vi "run_control.vi"() -> ()   [LabVIEW 2011]
panel:
  out "error out":errorcluster
  out "Last Remote Port":i64
  out "Last Remote Address":string
  out "Connection Msg":errorcluster
  out "Real-time Data from PLCs (Actuation)":string[][](array[string])
  out "# of data":i32
  out "# of data":i32
  out "# of data":i32
  out "# of data":i32
  out "# of received data":u64
  out "Real-time Data from People Counter":string[][](array[string])
  out "Real-time Data from PLCs (Sensing)":string[][](array[string])
  out "Real-time Data from Motes":string[][](array[string])
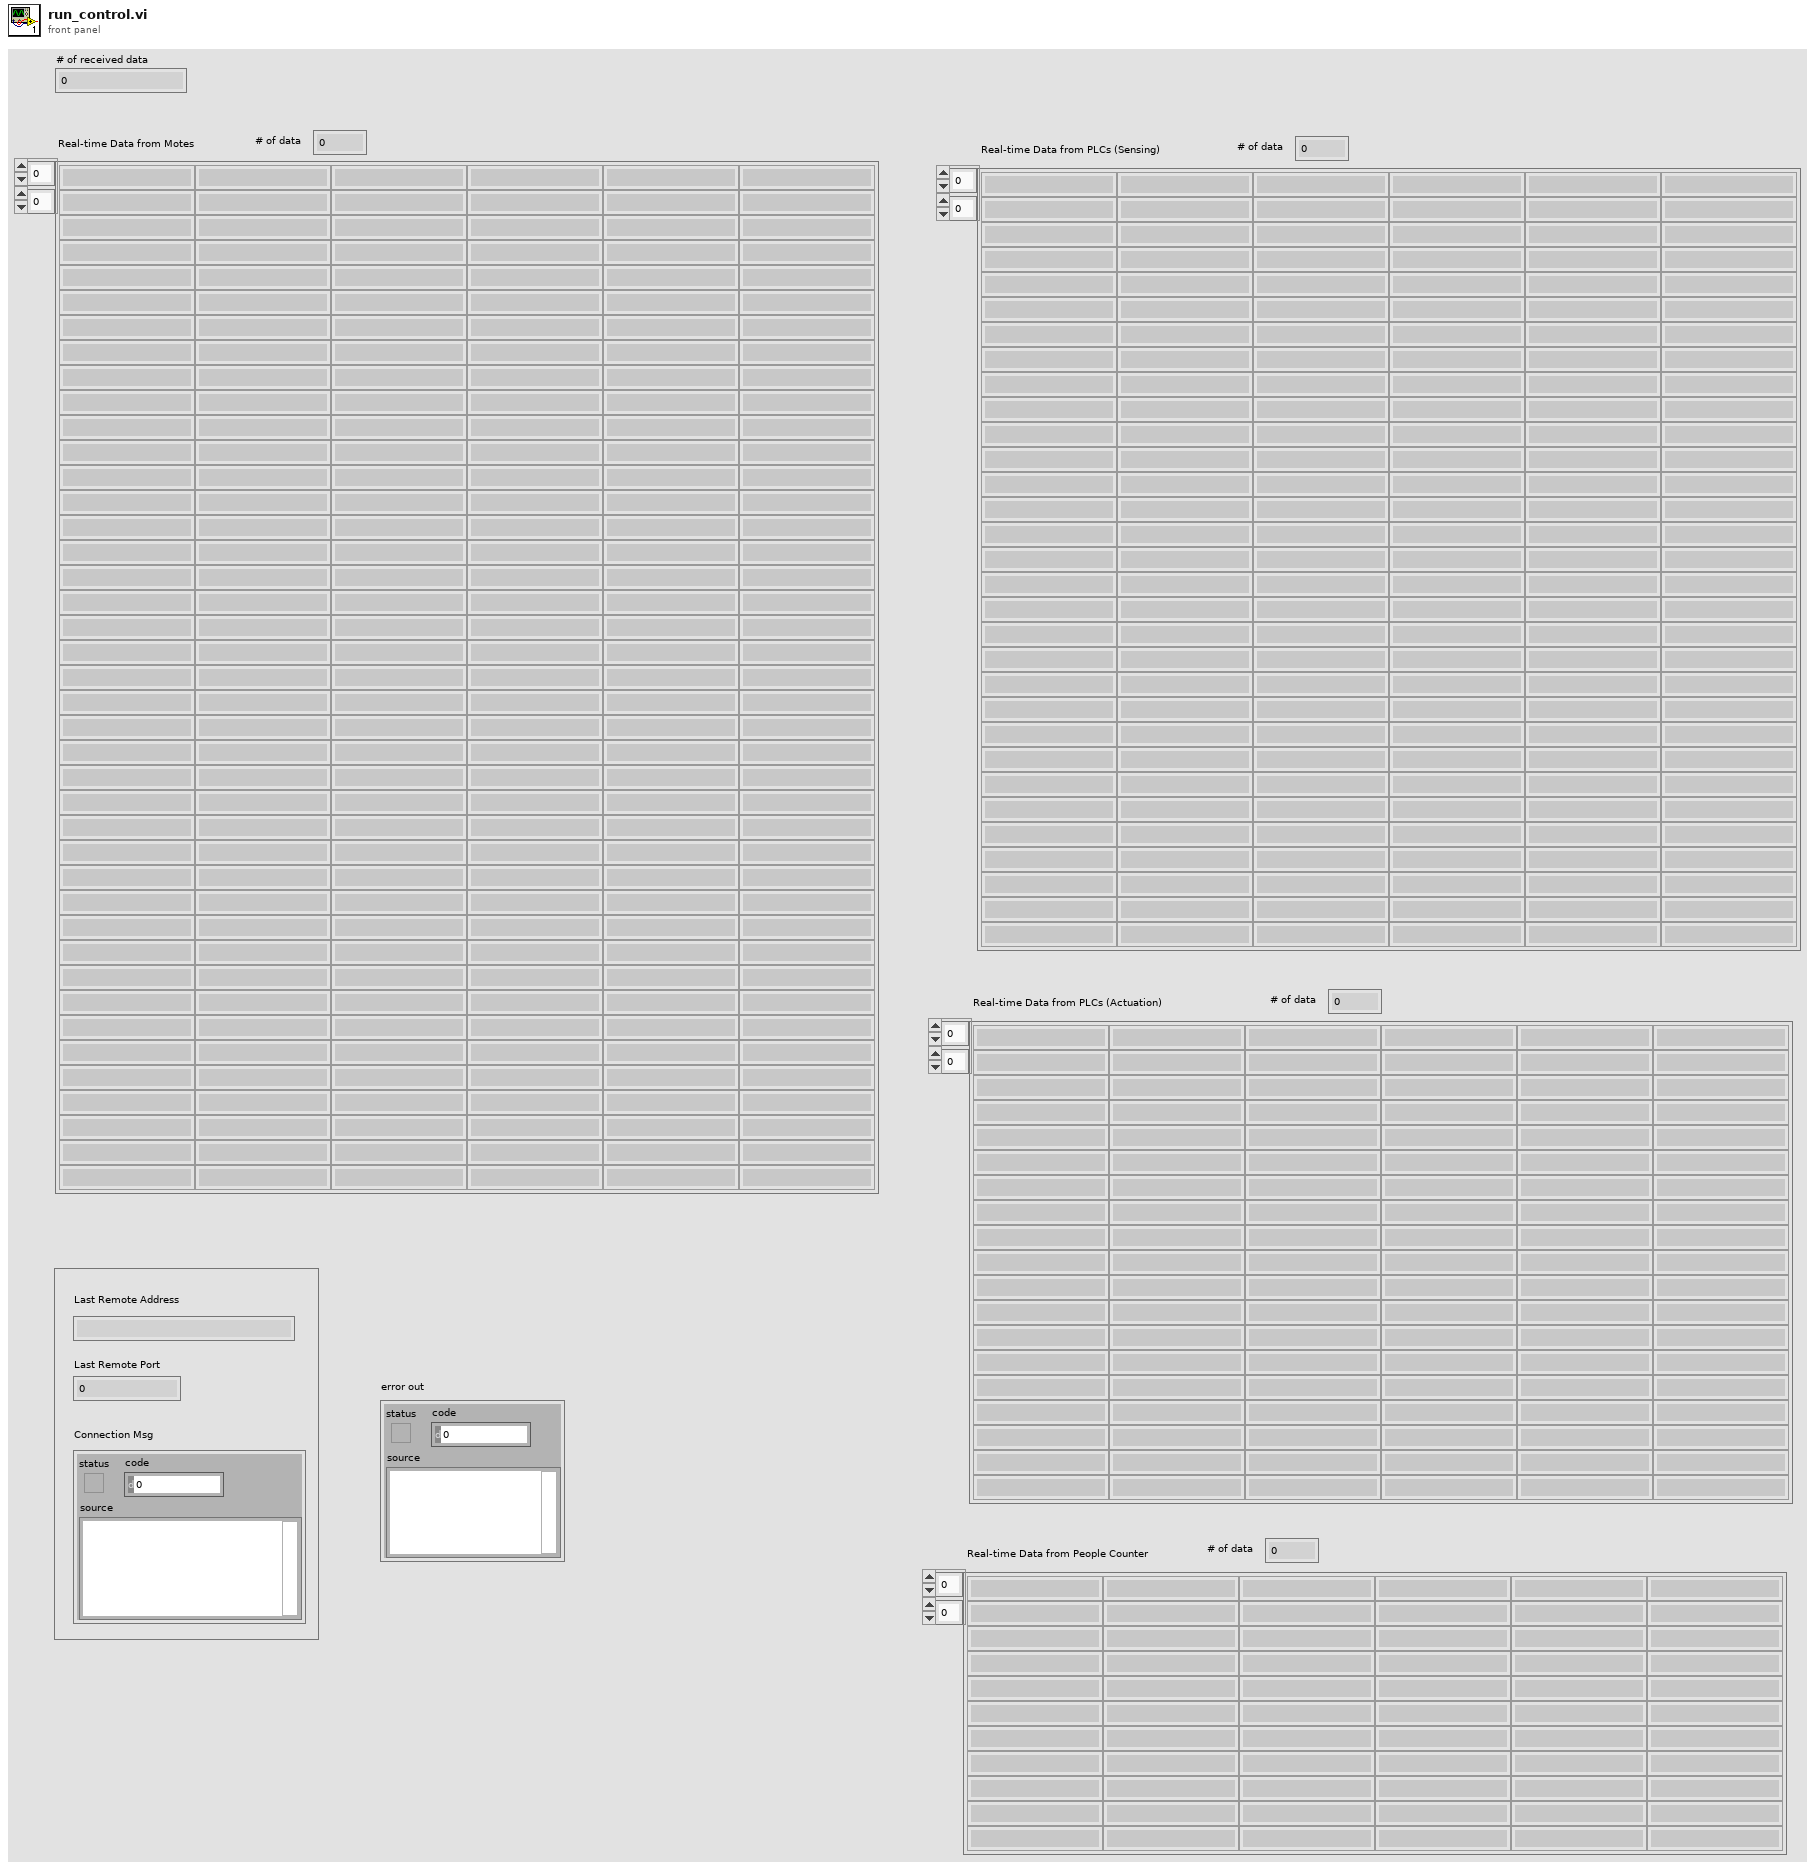
[diagram p1: front panel]
types:
  T1 = cluster{string, string, string, string, string, string}
  T2 = enum16{"Read", "Write", "ReadWrite", "BufferedRead", "BufferedReadWrite"}
  T3 = cluster{string, "output string":string, string, string, "date/time string":string, "output string":string}
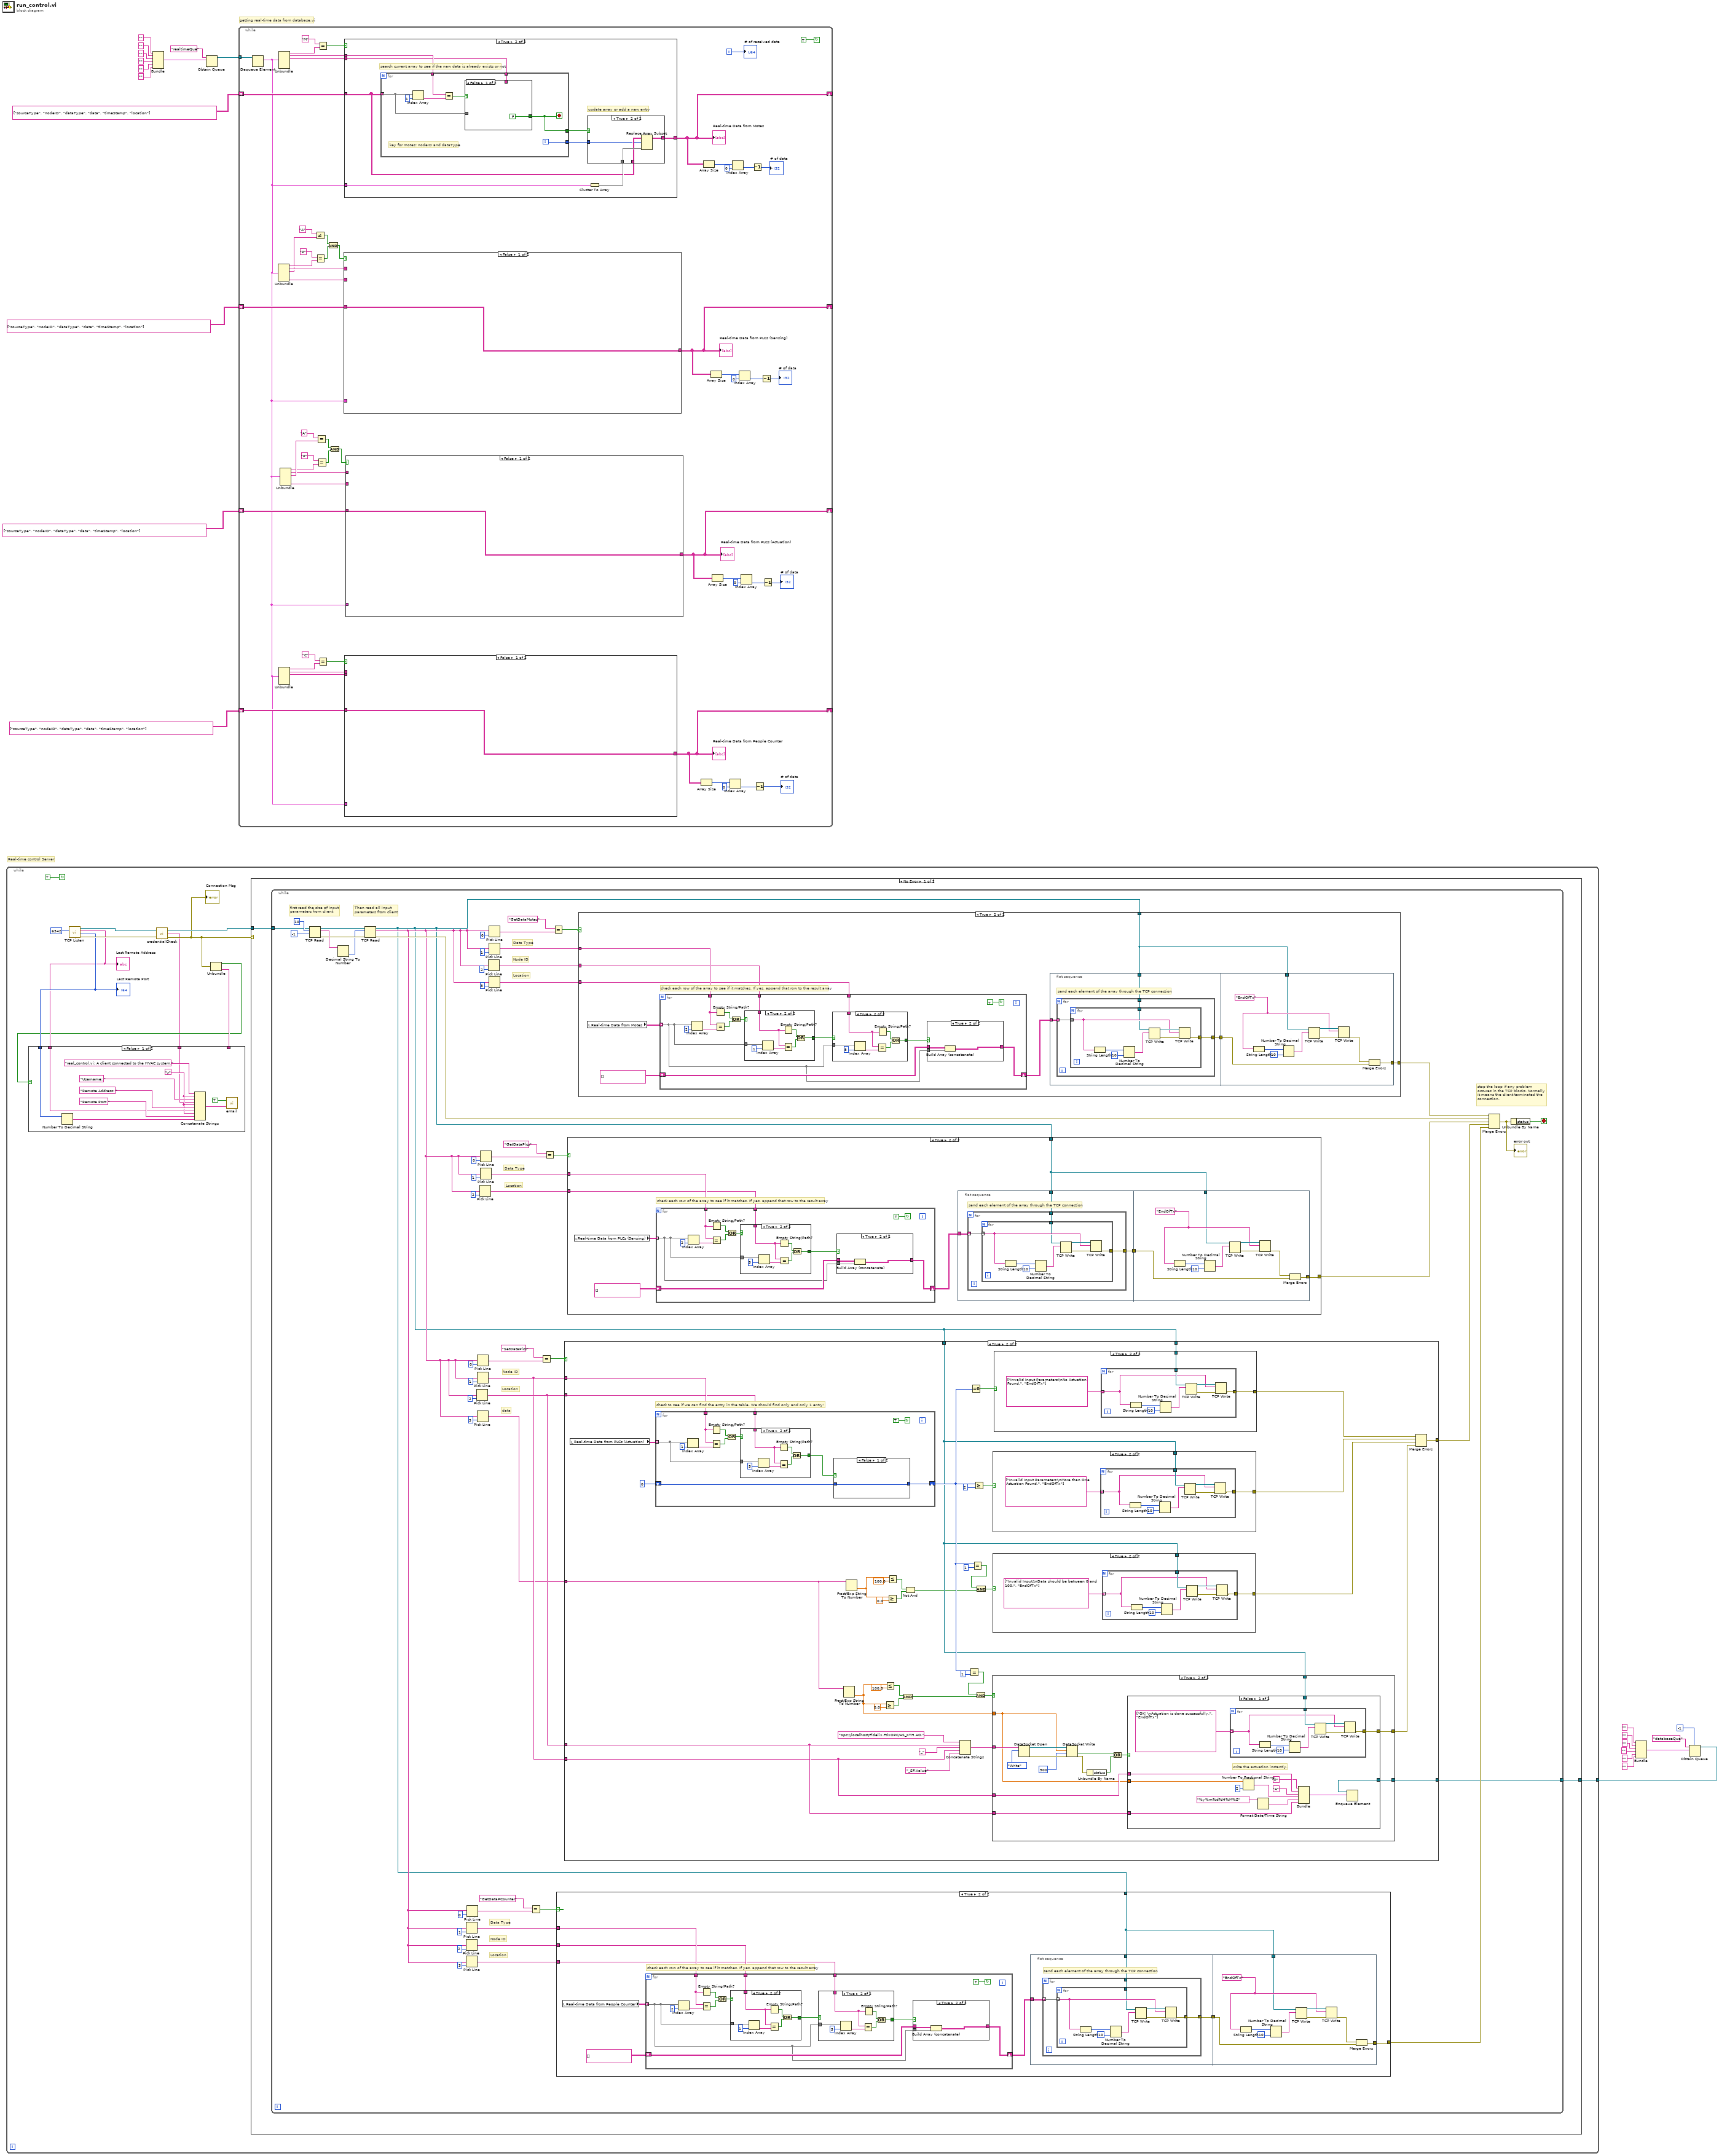
[diagram p0: block diagram]
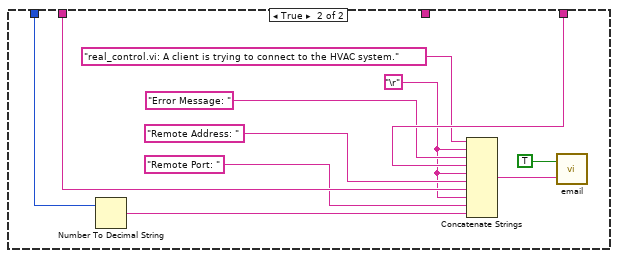
[diagram p2: hidden frame]
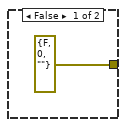
[diagram p3: hidden frame]
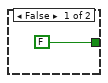
[diagram p5: hidden frame]
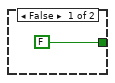
[diagram p6: hidden frame]
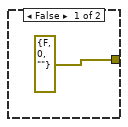
[diagram p7: hidden frame]
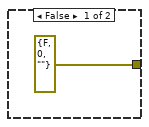
[diagram p8: hidden frame]
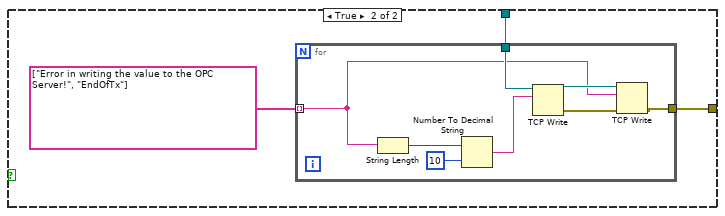
[diagram p9: hidden frame]
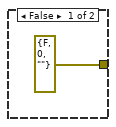
[diagram p10: hidden frame]
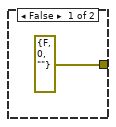
[diagram p11: hidden frame]
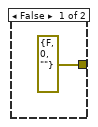
[diagram p12: hidden frame]
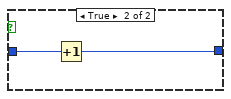
[diagram p13: hidden frame]
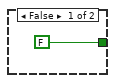
[diagram p14: hidden frame]
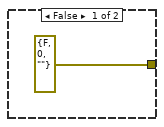
[diagram p15: hidden frame]
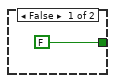
[diagram p17: hidden frame]
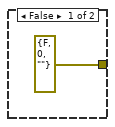
[diagram p18: hidden frame]
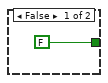
[diagram p20: hidden frame]
diagram:
  # "Real-time control Server"
  # "getting real-time data from database.vi"
  n1 = Bundle("", "", "", "", "", "") -> (w20:T1)  [unwired: 1 in]
  n2 = Obtain Queue(name (unnamed)="realtimeQue", element data type=w20) -> (queue out=w16:refnum<queue>)  [unwired: 3 in, 2 out]
  n3 = while {
    tunnel: w16 -> [w78]
    shift-right: [w54] -> _
    shift-left: string[][] [["sourceType", "nodeID", "dataType", "data", "timeStamp", "location"]] ("array") -> [w77]
    shift-right: [w59] -> _
    shift-left: string[][] [["sourceType", "nodeID", "dataType", "data", "timeStamp", "location"]] ("array") -> [w68]
    shift-right: [w51] -> _
    shift-left: string[][] [["sourceType", "nodeID", "dataType", "data", "timeStamp", "location"]] ("array") -> [w62]
    shift-right: [w25] -> _
    shift-left: string[][] [["sourceType", "nodeID", "dataType", "data", "timeStamp", "location"]] ("array") -> [w26]
    i -> [w60]
    stop <- TRUE continue-if-true
    n4 = Dequeue Element(queue=w78) -> (element=w24:T1)  [unwired: 2 in, 3 out]
    n5 = Unbundle(w24) -> (w70:string, w69:string, w44:string, w61:string)  [unwired: 2 out]
    n6 = Unbundle(w24) -> (w74:string, w76:string, w75:string)  [unwired: 3 out]
    n7 = Unbundle(w24) -> (w65:string, w63:string, w64:string)  [unwired: 3 out]
    n8 = Unbundle(w24) -> (w28:string, w29:string, w35:string, w30:string)  [unwired: 2 out]
    n9 = Not Equal?(x="A", y=w44) -> (x != y?=w42:bool)
    n10 = Equal?(x="P", y=w70) -> (x = y?=w41:bool)
    n11 = Equal?(x="A", y=w35) -> (x = y?=w37:bool)
    n12 = Equal?(x="P", y=w28) -> (x = y?=w38:bool)
    n13 = Equal?(x="M", y=w74) -> (x = y?=w72:bool)
    n14 = Equal?(x="C", y=w65) -> (x = y?=w67:bool)
    n15 = And(x=w42, y=w41) -> (x .and. y?=w40:bool)
    n16 = And(x=w37, y=w38) -> (x .and. y?=w39:bool)
    n17 = case shown="False" w40 {
      tunnel: w24 -> [_ w152]
      tunnel: w68 -> [w144 w147]
      tunnel: [w144 w148] -> w59
      tunnel: w69 -> [_ w146]
      tunnel: w61 -> [_ w145]
      frame False {
      }
      frame True {
        # "search current array to see if the new data is already exists or not"
        # "update array or add a new entry"
        n18 = for {
          tunnel: w147 -> [w163] mode=indexing
          tunnel: w146 -> [w167]
          tunnel: [w162] -> w151
          tunnel: [w166] -> w150
          tunnel: w145 -> [w164]
          i -> [w166]
          stop <- w162 stop-if-true
          # "key for plcs: nodeID and location"
          n19 = Index Array(array=w163, index=1) -> (element=w168:string)
          n20 = Equal?(x=w167, y=w168) -> (x = y?=w165:bool)
          n21 = case shown="True" w165 {
            tunnel: w163 -> [_ w174]
            tunnel: w164 -> [_ w172]
            tunnel: [FALSE w171] -> w162
            frame False {
            }
            frame True {
              n22 = Index Array(array=w174, index=5) -> (element=w173:string)
              n23 = Equal?(x=w172, y=w173) -> (x = y?=w171:bool)
            }
          }
        }
        n24 = Cluster To Array(cluster=w152) -> (array=w149:string[])
        n25 = case shown="True" w151 {
          tunnel: w147 -> [w157 w159]
          tunnel: w150 -> [w154 w158]
          tunnel: w149 -> [w156 w160]
          tunnel: [w155 w161] -> w148
          frame False {
            n26 = Increment(x=w154) -> (x+1=w153:i32)
            n27 = Insert Into Array(array=w157, index (row)=w153, new element=w156) -> (w155:string[][])  [unwired: 1 in]
          }
          frame True {
            n28 = Replace Array Subset(array=w159, new element=w160, index (row)=w158) -> (w161:string[][])  [unwired: 1 in]
          }
        }
      }
    }
    "Real-time Data from PLCs (Sensing)" <- w59
    n29 = case shown="True" w72 {
      tunnel: w24 -> [_ w184]
      tunnel: w77 -> [w176 w178]
      tunnel: [w176 w179] -> w54
      tunnel: w76 -> [_ w183]
      tunnel: w75 -> [_ w177]
      frame False {
      }
      frame True {
        # "update array or add a new entry"
        # "search current array to see if the new data is already exists or not"
        n30 = for {
          tunnel: w178 -> [w196] mode=indexing
          tunnel: w183 -> [w199]
          tunnel: [w194] -> w182
          tunnel: [w198] -> w181
          tunnel: w177 -> [w195]
          i -> [w198]
          stop <- w194 stop-if-true
          # "key for motes: nodeID and dataType"
          n31 = Index Array(array=w196, index=1) -> (element=w200:string)
          n32 = Equal?(x=w199, y=w200) -> (x = y?=w197:bool)
          n33 = case shown="False" w197 {
            tunnel: w196 -> [_ w206]
            tunnel: w195 -> [_ w204]
            tunnel: [FALSE w203] -> w194
            frame False {
            }
            frame True {
              n34 = Index Array(array=w206, index=2) -> (element=w205:string)
              n35 = Equal?(x=w204, y=w205) -> (x = y?=w203:bool)
            }
          }
        }
        n36 = Cluster To Array(cluster=w184) -> (array=w180:string[])
        n37 = case shown="True" w182 {
          tunnel: w178 -> [w189 w191]
          tunnel: w181 -> [w186 w190]
          tunnel: w180 -> [w188 w192]
          tunnel: [w187 w193] -> w179
          frame False {
            n38 = Increment(x=w186) -> (x+1=w185:i32)
            n39 = Insert Into Array(array=w189, index (row)=w185, new element=w188) -> (w187:string[][])  [unwired: 1 in]
          }
          frame True {
            n40 = Replace Array Subset(array=w191, new element=w192, index (row)=w190) -> (w193:string[][])  [unwired: 1 in]
          }
        }
      }
    }
    "Real-time Data from Motes" <- w54
    n41 = case shown="False" w67 {
      tunnel: w24 -> [_ w120]
      tunnel: w62 -> [w112 w114]
      tunnel: [w112 w115] -> w51
      tunnel: w63 -> [_ w119]
      tunnel: w64 -> [_ w113]
      frame False {
      }
      frame True {
        # "update array or add a new entry"
        # "search current array to see if the new data is already exists or not"
        n42 = for {
          tunnel: w114 -> [w132] mode=indexing
          tunnel: w119 -> [w135]
          tunnel: [w130] -> w118
          tunnel: [w134] -> w117
          tunnel: w113 -> [w131]
          i -> [w134]
          stop <- w130 stop-if-true
          # "key for counter: nodeID and dataType"
          n43 = Index Array(array=w132, index=1) -> (element=w136:string)
          n44 = Equal?(x=w135, y=w136) -> (x = y?=w133:bool)
          n45 = case shown="True" w133 {
            tunnel: w132 -> [_ w142]
            tunnel: w131 -> [_ w140]
            tunnel: [FALSE w139] -> w130
            frame False {
            }
            frame True {
              n46 = Index Array(array=w142, index=2) -> (element=w141:string)
              n47 = Equal?(x=w140, y=w141) -> (x = y?=w139:bool)
            }
          }
        }
        n48 = Cluster To Array(cluster=w120) -> (array=w116:string[])
        n49 = case shown="True" w118 {
          tunnel: w114 -> [w125 w127]
          tunnel: w117 -> [w122 w126]
          tunnel: w116 -> [w124 w128]
          tunnel: [w123 w129] -> w115
          frame False {
            n50 = Increment(x=w122) -> (x+1=w121:i32)
            n51 = Insert Into Array(array=w125, index (row)=w121, new element=w124) -> (w123:string[][])  [unwired: 1 in]
          }
          frame True {
            n52 = Replace Array Subset(array=w127, new element=w128, index (row)=w126) -> (w129:string[][])  [unwired: 1 in]
          }
        }
      }
    }
    "Real-time Data from People Counter" <- w51
    n53 = case shown="False" w39 {
      tunnel: w24 -> [_ w88]
      tunnel: w26 -> [w80 w83]
      tunnel: [w80 w84] -> w25
      tunnel: w29 -> [_ w82]
      tunnel: w30 -> [_ w81]
      frame False {
      }
      frame True {
        # "search current array to see if the new data is already exists or not"
        # "update array or add a new entry"
        n54 = for {
          tunnel: w83 -> [w99] mode=indexing
          tunnel: w82 -> [w103]
          tunnel: [w98] -> w87
          tunnel: [w102] -> w86
          tunnel: w81 -> [w100]
          i -> [w102]
          stop <- w98 stop-if-true
          # "key for plcs: nodeID and location"
          n55 = Index Array(array=w99, index=1) -> (element=w104:string)
          n56 = Equal?(x=w103, y=w104) -> (x = y?=w101:bool)
          n57 = case shown="True" w101 {
            tunnel: w99 -> [_ w110]
            tunnel: w100 -> [_ w108]
            tunnel: [FALSE w107] -> w98
            frame False {
            }
            frame True {
              n58 = Index Array(array=w110, index=5) -> (element=w109:string)
              n59 = Equal?(x=w108, y=w109) -> (x = y?=w107:bool)
            }
          }
        }
        n60 = Cluster To Array(cluster=w88) -> (array=w85:string[])
        n61 = case shown="False" w87 {
          tunnel: w83 -> [w93 w95]
          tunnel: w86 -> [w90 w94]
          tunnel: w85 -> [w92 w96]
          tunnel: [w91 w97] -> w84
          frame False {
            n62 = Increment(x=w90) -> (x+1=w89:i32)
            n63 = Insert Into Array(array=w93, index (row)=w89, new element=w92) -> (w91:string[][])  [unwired: 1 in]
          }
          frame True {
            n64 = Replace Array Subset(array=w95, new element=w96, index (row)=w94) -> (w97:string[][])  [unwired: 1 in]
          }
        }
      }
    }
    "Real-time Data from PLCs (Actuation)" <- w25
    n65 = Array Size(array=w51) -> (size(s)=w52:i32[])
    n66 = Array Size(array=w54) -> (size(s)=w55:i32[])
    n67 = Array Size(array=w59) -> (size(s)=w58:i32[])
    n68 = Array Size(array=w25) -> (size(s)=w31:i32[])
    n69 = Index Array(array=w52, index=0) -> (element=w46:i32)
    n70 = Index Array(array=w55, index=0) -> (element=w50:i32)
    n71 = Index Array(array=w58, index=0) -> (element=w48:i32)
    n72 = Index Array(array=w31, index=0) -> (element=w33:i32)
    n73 = Decrement(x=w50) -> (x-1=→"# of data":i32)
    n74 = Decrement(x=w46) -> (x-1=→"# of data":i32)
    n75 = Decrement(x=w48) -> (x-1=→"# of data":i32)
    n76 = Decrement(x=w33) -> (x-1=→"# of data":i32)
    "# of received data" <- w60
  }
  n77 = Bundle("", "", "", "", "", "") -> (w6:T1)  [unwired: 1 in]
  n78 = Obtain Queue(max queue size (-1, unlimited)=-1, name (unnamed)="databaseQue", element data type=w6) -> (queue out=w1:refnum<queue>)  [unwired: 2 in, 2 out]
  n79 = while {
    tunnel: w1 -> [w211]
    stop <- TRUE continue-if-true
    n80 = call <vilib>:"TCP Listen.vi"("port"=u16 6342) -> ("error out"=w217:errorcluster, "remote port"=w214:u16, "remote address"=w210:string, "connection ID"=w216:refnum<k5>)  [unwired: 6 in, 1 out]
    "Last Remote Address" <- w210
    "Last Remote Port" <- w214
    n81 = call "credentialCheck.vi"("connection ID in"=w216, "error in"=w217) -> ("connection ID out"=w215:refnum<k5>, "user"=w208:string, "error out"=w213:errorcluster)
    "Connection Msg" <- w213
    n82 = Unbundle(w213) -> ("status"=w209:bool, "source"=w212:string)  [unwired: 1 out]
    n83 = case shown="False" w209 {
      tunnel: w214 -> [w221 w239]
      tunnel: w212 -> [_ w238]
      tunnel: w210 -> [w222 w234]
      tunnel: w208 -> [w220 _]
      frame False {
        w225 = "\r"
        n84 = Number To Decimal String(number=w221) -> (decimal integer string=w223:string)  [unwired: 1 in]
        n85 = Concatenate Strings("real_control.vi: A client connected to the HVAC system.", w225, "Username: ", w220, w225, "Remote Address: ", w222, w225, "Remote Port: ", w223) -> (w230:string)
        n86 = call "email.vi"("Body"=w230, "Enable"=TRUE) -> ()  [unwired: 1 in]
      }
      frame True {
        w233 = "\r"
        n87 = Number To Decimal String(number=w239) -> (decimal integer string=w231:string)  [unwired: 1 in]
        n88 = Concatenate Strings("real_control.vi: A client is trying to connect to the HVAC system.", w233, "Error Message: ", w238, w233, "Remote Address: ", w234, w233, "Remote Port: ", w231) -> (w241:string)
        n89 = call "email.vi"("Body"=w241, "Enable"=TRUE) -> ()  [unwired: 1 in]
      }
    }
    n90 = case shown="No Error" w213 {
      tunnel: w215 -> [w243 _]
      tunnel: w211 -> [w242 _]
      frame No Error {
        n91 = while {
          tunnel: w243 -> [w293]
          tunnel: w242 -> [w245]
          stop <- w285 stop-if-true
          # "Location"
          # "Node ID"
          # "Data Type"
          # "data"
          # "stop the loop if any problem\noccures in the TCP blocks. Normally\nit means the client terminated the\nconnection."
          # "Location"
          # "Node ID"
          # "Location"
          # "Data Type"
          # "Then read all input \nparameters from client"
          # "Location"
          # "Node ID"
          # "Data Type"
          # "first read the size of input \nparameters from client"
          n92 = TCP Read(connection ID=w293, bytes to read=10, 9:-1 ("timeout ms (25000)")) -> (connection ID out=w289:refnum<k5>, data out=w290:string, error out=w288:errorcluster)  [unwired: 2 in]
          n93 = Decimal String To Number(string=w290) -> (number=w287:i32)  [unwired: 2 in, 1 out]
          n94 = TCP Read(connection ID=w289, bytes to read=w287, error in (no error)=w288) -> (connection ID out=w247:refnum<k5>, data out=w248:string, error out=w279:errorcluster)  [unwired: 2 in]
          n95 = Pick Line(multi-line string=w248, line index=2) -> (output string=w257:string)  [unwired: 1 in]
          n96 = Pick Line(multi-line string=w248, line index=1) -> (output string=w256:string)  [unwired: 1 in]
          n97 = Pick Line(multi-line string=w248, line index=3) -> (output string=w258:string)  [unwired: 1 in]
          n98 = Pick Line(multi-line string=w248, line index=0) -> (output string=w255:string)  [unwired: 1 in]
          n99 = Pick Line(multi-line string=w248, line index=2) -> (output string=w263:string)  [unwired: 1 in]
          n100 = Pick Line(multi-line string=w248, line index=1) -> (output string=w262:string)  [unwired: 1 in]
          n101 = Pick Line(multi-line string=w248, line index=3) -> (output string=w260:string)  [unwired: 1 in]
          n102 = Pick Line(multi-line string=w248, line index=0) -> (output string=w264:string)  [unwired: 1 in]
          n103 = Pick Line(multi-line string=w248, line index=2) -> (output string=w278:string)  [unwired: 1 in]
          n104 = Pick Line(multi-line string=w248, line index=1) -> (output string=w277:string)  [unwired: 1 in]
          n105 = Pick Line(multi-line string=w248, line index=0) -> (output string=w276:string)  [unwired: 1 in]
          n106 = Pick Line(multi-line string=w248, line index=2) -> (output string=w282:string)  [unwired: 1 in]
          n107 = Pick Line(multi-line string=w248, line index=1) -> (output string=w283:string)  [unwired: 1 in]
          n108 = Pick Line(multi-line string=w248, line index=3) -> (output string=w281:string)  [unwired: 1 in]
          n109 = Pick Line(multi-line string=w248, line index=0) -> (output string=w284:string)  [unwired: 1 in]
          n110 = Equal?(x="GetDataPCounter", y=w255) -> (x = y?=w253:bool)
          n111 = Equal?(x="SetDataPlcs", y=w264) -> (x = y?=w266:bool)
          n112 = Equal?(x="GetDataPlcs", y=w276) -> (x = y?=w274:bool)
          n113 = Equal?(x="GetDataMotes", y=w284) -> (x = y?=w292:bool)
          n114 = case shown="True" w253 {
            tunnel: w256 -> [_ w308]
            tunnel: w257 -> [_ w307]
            tunnel: w258 -> [_ w306]
            tunnel: w247 -> [_ w300]
            tunnel: [errorcluster {"status"=FALSE, "code"=0, "source"=""} ("error IO") w301] -> w246
            frame False {
            }
            frame True {
              # "check each row of the array to see if it matches. If yes, append that row to the result array"
              n115 = local read "Real-time Data from People Counter"() -> (w303:string[][])
              n116 = for {
                tunnel: w303 -> [w333] mode=indexing
                tunnel: w308 -> [w339]
                tunnel: w307 -> [w344]
                tunnel: w306 -> [w343]
                shift-right: [w341] -> w304
                shift-left: string[][] [] -> [w334]
                stop <- TRUE continue-if-true
                n117 = Index Array(array=w333, index=2) -> (element=w345:string)
                n118 = Empty String/Path?(string/path=w339) -> (empty?=w337:bool)
                n119 = Equal?(x=w339, y=w345) -> (x = y?=w338:bool)
                n120 = Or(x=w337, y=w338) -> (x .or. y?=w336:bool)
                n121 = case shown="True" w336 {
                  tunnel: w333 -> [_ w365]
                  tunnel: w344 -> [_ w360]
                  tunnel: [FALSE w363] -> w335
                  frame False {
                  }
                  frame True {
                    n122 = Index Array(array=w365, index=1) -> (element=w364:string)
                    n123 = Empty String/Path?(string/path=w360) -> (empty?=w361:bool)
                    n124 = Equal?(x=w360, y=w364) -> (x = y?=w362:bool)
                    n125 = Or(x=w361, y=w362) -> (x .or. y?=w363:bool)
                  }
                }
                n126 = case shown="True" w335 {
                  tunnel: w333 -> [_ w357]
                  tunnel: w343 -> [_ w353]
                  tunnel: [FALSE w352] -> w342
                  frame False {
                  }
                  frame True {
                    n127 = Index Array(array=w357, index=5) -> (element=w356:string)
                    n128 = Equal?(x=w353, y=w356) -> (x = y?=w355:bool)
                    n129 = Empty String/Path?(string/path=w353) -> (empty?=w354:bool)
                    n130 = Or(x=w354, y=w355) -> (x .or. y?=w352:bool)
                  }
                }
                n131 = case shown="True" w342 {
                  tunnel: w334 -> [w347 w350]
                  tunnel: w333 -> [_ w349]
                  tunnel: [w347 w348] -> w341
                  frame False {
                  }
                  frame True {
                    n132 = Build Array (concatenate)(w350, w349) -> (w348:string[][])
                  }
                }
              }
              n133 = flat-sequence {
                tunnel: w304 -> [w311]
                tunnel: w300 -> [w310]
                tunnel: [w309] -> w302
                tunnel: w302 -> [w325]
                tunnel: [w324] -> w301
                tunnel: w300 -> [w323]
                frame #0 {
                  # "send each element of the array through the TCP connection"
                  n134 = for {
                    tunnel: w311 -> [w314] mode=indexing
                    tunnel: w310 -> [w313]
                    tunnel: [w312] -> w309
                    n135 = for {
                      tunnel: w314 -> [w317] mode=indexing
                      tunnel: w313 -> [w316]
                      tunnel: [w315] -> w312
                      n136 = String Length(string=w317) -> (length=w321:i32)
                      n137 = Number To Decimal String(number=w321, width (-)=i16 10) -> (decimal integer string=w320:string)
                      n138 = TCP Write(connection ID=w316, data in=w320) -> (connection ID out=w318:refnum<k5>, error out=w319:errorcluster)  [unwired: 2 in, 1 out]
                      n139 = TCP Write(connection ID=w318, data in=w317, error in (no error)=w319) -> (error out=w315:errorcluster)  [unwired: 1 in, 2 out]
                    }
                  }
                }
                frame #1 {
                  w327 = "EndOfTx" ("data in")
                  n140 = String Length(string=w327) -> (length=w330:i32)
                  n141 = Number To Decimal String(number=w330, width (-)=i16 10) -> (decimal integer string=w331:string)
                  n142 = TCP Write(connection ID=w323, data in=w331) -> (connection ID out=w328:refnum<k5>, error out=w332:errorcluster)  [unwired: 2 in, 1 out]
                  n143 = TCP Write(connection ID=w328, data in=w327, error in (no error)=w332) -> (error out=w326:errorcluster)  [unwired: 1 in, 2 out]
                  n144 = Merge Errors(w326, w325) -> (w324:errorcluster)
                }
              }
            }
          }
          n145 = case shown="True" w266 {
            tunnel: w262 -> [_ w408]
            tunnel: w263 -> [_ w407]
            tunnel: w247 -> [_ w406]
            tunnel: w247 -> [_ w386]
            tunnel: w263 -> [_ w369]
            tunnel: w262 -> [_ w368]
            tunnel: w260 -> [_ w373]
            tunnel: [errorcluster {"status"=FALSE, "code"=0, "source"=""} ("error IO") w372] -> w259
            tunnel: w245 -> [_ w370]
            frame False {
            }
            frame True {
              # "check to see if we can find the entry in the table. We should find only and only 1 entry!"
              n146 = local read "Real-time Data from PLCs (Actuation)"() -> (w405:string[][])
              n147 = for {
                tunnel: w405 -> [w496] mode=indexing
                tunnel: w408 -> [w500]
                tunnel: w407 -> [w503]
                shift-right: [w502] -> w387
                shift-left: u64 0 -> [w494]
                stop <- TRUE continue-if-true
                n148 = Index Array(array=w496, index=1) -> (element=w504:string)
                n149 = Empty String/Path?(string/path=w500) -> (empty?=w498:bool)
                n150 = Equal?(x=w500, y=w504) -> (x = y?=w499:bool)
                n151 = Or(x=w498, y=w499) -> (x .or. y?=w497:bool)
                n152 = case shown="True" w497 {
                  tunnel: w496 -> [_ w515]
                  tunnel: w503 -> [_ w510]
                  tunnel: [FALSE w513] -> w495
                  frame False {
                  }
                  frame True {
                    n153 = Index Array(array=w515, index=5) -> (element=w514:string)
                    n154 = Empty String/Path?(string/path=w510) -> (empty?=w511:bool)
                    n155 = Equal?(x=w510, y=w514) -> (x = y?=w512:bool)
                    n156 = Or(x=w511, y=w512) -> (x .or. y?=w513:bool)
                  }
                }
                n157 = case shown="False" w495 {
                  tunnel: [w506 w507] -> w502
                  tunnel: w494 -> [w506 w508]
                  frame False {
                  }
                  frame True {
                    n158 = Increment(x=w508) -> (x+1=w507:u64)
                  }
                }
              }
              n159 = Fract/Exp String To Number(string=w373) -> (number=w374:dbl)  [unwired: 3 in, 1 out]
              n160 = Fract/Exp String To Number(string=w373) -> (number=w380:dbl)  [unwired: 3 in, 1 out]
              n161 = Greater Or Equal?(x=w374, y=0.0) -> (x >= y?=w379:bool)
              n162 = Less Or Equal?(x=w374, y=100.0) -> (x <= y?=w378:bool)
              n163 = Greater Or Equal?(x=w380, y=0.0) -> (x >= y?=w382:bool)
              n164 = Less Or Equal?(x=w380, y=100.0) -> (x <= y?=w383:bool)
              n165 = And(x=w378, y=w379) -> (x .and. y?=w375:bool)
              n166 = Not And(1:w382, 2:w383) -> (0:w381:bool)
              n167 = Concatenate Strings("opc://localhost/Fidelix.FdxOPC/AS_KTH.AO.", w369, "_", w368, "_SF.Value") -> (w397:string)
              n168 = Equal?(x=w387, y=u64 1) -> (x = y?=w390:bool)
              n169 = Equal To 0?(x=w387) -> (x = 0?=w403:bool)
              n170 = Equal?(x=w387, y=u64 1) -> (x = y?=w393:bool)
              n171 = Greater Or Equal?(x=w387, y=u64 2) -> (x >= y?=w399:bool)
              n172 = And(x=w390, y=w375) -> (x .and. y?=w388:bool)
              n173 = And(x=w393, y=w381) -> (x .and. y?=w392:bool)
              n174 = case shown="True" w388 {
                tunnel: w386 -> [_ w419]
                tunnel: w397 -> [_ w420]
                tunnel: w374 -> [_ w410]
                tunnel: [errorcluster {"status"=FALSE, "code"=0, "source"=""} ("error out") w418] -> w371
                tunnel: w370 -> [_ w413]
                tunnel: w369 -> [_ w412]
                tunnel: w368 -> [_ w411]
                frame False {
                }
                frame True {
                  n175 = DataSocket Open(10:T2."Write" ("mode"), 11:w420) -> (0:w424:errorcluster, 3:w423:refnum<k13>)  [unwired: 1 in, 1 out]
                  n176 = DataSocket Write(8:w424, 9:500 ("ms timeout (10000)"), 10:w410, 11:w423) -> (0:w416:errorcluster, 1:w415:bool)  [unwired: 1 out]
                  n177 = Unbundle By Name(w416) -> ("status"=w417:bool)
                  n178 = Or(x=w415, y=w417) -> (x .or. y?=w414:bool)
                  n179 = case shown="False" w414 {
                    tunnel: w419 -> [w437 w449]
                    tunnel: [w436 w447] -> w418
                    tunnel: w413 -> [w433 _]
                    tunnel: w412 -> [w430 _]
                    tunnel: w411 -> [w429 _]
                    tunnel: w410 -> [w427 _]
                    frame False {
                      # "write the actuation instantly."
                      n180 = for {
                        tunnel: w437 -> [w446]
                        tunnel: string[] ["OK! \nActuation is done successfully.", "EndOfTx"] -> [w440] mode=indexing
                        tunnel: [w439] -> w436
                        n181 = String Length(string=w440) -> (length=w444:i32)
                        n182 = Number To Decimal String(number=w444, width (-)=i16 10) -> (decimal integer string=w443:string)
                        n183 = TCP Write(connection ID=w446, data in=w443) -> (connection ID out=w441:refnum<k5>, error out=w442:errorcluster)  [unwired: 2 in, 1 out]
                        n184 = TCP Write(connection ID=w441, data in=w440, error in (no error)=w442) -> (error out=w439:errorcluster)  [unwired: 1 in, 2 out]
                      }
                      n185 = Number To Fractional String(number=w427, precision (6)=i16 2) -> (F-format string=w426:string)  [unwired: 2 in]
                      n186 = Format Date/Time String(time format string (%c)="%y%m%d%H%M%S") -> (date/time string=w431:string)  [unwired: 2 in]
                      n187 = Bundle("P", "output string"=w429, "A", w426, "date/time string"=w431, "output string"=w430) -> (w434:T3)  [unwired: 1 in]
                      n188 = Enqueue Element(queue=w433, element=w434) -> ()  [unwired: 2 in, 3 out]
                    }
                    frame True {
                      n189 = for {
                        tunnel: w449 -> [w457]
                        tunnel: string[] ["Error in writing the value to the OPC Server!", "EndOfTx"] -> [w451] mode=indexing
                        tunnel: [w450] -> w447
                        n190 = String Length(string=w451) -> (length=w455:i32)
                        n191 = Number To Decimal String(number=w455, width (-)=i16 10) -> (decimal integer string=w454:string)
                        n192 = TCP Write(connection ID=w457, data in=w454) -> (connection ID out=w452:refnum<k5>, error out=w453:errorcluster)  [unwired: 2 in, 1 out]
                        n193 = TCP Write(connection ID=w452, data in=w451, error in (no error)=w453) -> (error out=w450:errorcluster)  [unwired: 1 in, 2 out]
                      }
                    }
                  }
                }
              }
              n194 = case shown="True" w392 {
                tunnel: w386 -> [_ w461]
                tunnel: [errorcluster {"status"=FALSE, "code"=0, "source"=""} ("error out") w459] -> w391
                frame False {
                }
                frame True {
                  n195 = for {
                    tunnel: w461 -> [w469]
                    tunnel: string[] ["Invalid Input!\nData should be between 0 and 100.", "EndOfTx"] -> [w463] mode=indexing
                    tunnel: [w462] -> w459
                    n196 = String Length(string=w463) -> (length=w467:i32)
                    n197 = Number To Decimal String(number=w467, width (-)=i16 10) -> (decimal integer string=w466:string)
                    n198 = TCP Write(connection ID=w469, data in=w466) -> (connection ID out=w464:refnum<k5>, error out=w465:errorcluster)  [unwired: 2 in, 1 out]
                    n199 = TCP Write(connection ID=w464, data in=w463, error in (no error)=w465) -> (error out=w462:errorcluster)  [unwired: 1 in, 2 out]
                  }
                }
              }
              n200 = case shown="True" w399 {
                tunnel: w386 -> [_ w473]
                tunnel: [errorcluster {"status"=FALSE, "code"=0, "source"=""} ("error out") w471] -> w398
                frame False {
                }
                frame True {
                  n201 = for {
                    tunnel: w473 -> [w481]
                    tunnel: string[] ["Invalid Input Parameters!\nMore than One Actuation Found.", "EndOfTx"] -> [w475] mode=indexing
                    tunnel: [w474] -> w471
                    n202 = String Length(string=w475) -> (length=w479:i32)
                    n203 = Number To Decimal String(number=w479, width (-)=i16 10) -> (decimal integer string=w478:string)
                    n204 = TCP Write(connection ID=w481, data in=w478) -> (connection ID out=w476:refnum<k5>, error out=w477:errorcluster)  [unwired: 2 in, 1 out]
                    n205 = TCP Write(connection ID=w476, data in=w475, error in (no error)=w477) -> (error out=w474:errorcluster)  [unwired: 1 in, 2 out]
                  }
                }
              }
              n206 = case shown="True" w403 {
                tunnel: w406 -> [_ w485]
                tunnel: [errorcluster {"status"=FALSE, "code"=0, "source"=""} ("error out") w483] -> w401
                frame False {
                }
                frame True {
                  n207 = for {
                    tunnel: w485 -> [w493]
                    tunnel: string[] ["Invalid Input Parameters!\nNo Actuation Found.", "EndOfTx"] -> [w487] mode=indexing
                    tunnel: [w486] -> w483
                    n208 = String Length(string=w487) -> (length=w491:i32)
                    n209 = Number To Decimal String(number=w491, width (-)=i16 10) -> (decimal integer string=w490:string)
                    n210 = TCP Write(connection ID=w493, data in=w490) -> (connection ID out=w488:refnum<k5>, error out=w489:errorcluster)  [unwired: 2 in, 1 out]
                    n211 = TCP Write(connection ID=w488, data in=w487, error in (no error)=w489) -> (error out=w486:errorcluster)  [unwired: 1 in, 2 out]
                  }
                }
              }
              n212 = Merge Errors(w401, w398, w391, w371) -> (w372:errorcluster)
            }
          }
          n213 = case shown="True" w274 {
            tunnel: w277 -> [_ w525]
            tunnel: w278 -> [_ w524]
            tunnel: w247 -> [_ w518]
            tunnel: [errorcluster {"status"=FALSE, "code"=0, "source"=""} ("error IO") w520] -> w270
            frame False {
            }
            frame True {
              # "check each row of the array to see if it matches. If yes, append that row to the result array"
              n214 = local read "Real-time Data from PLCs (Sensing)"() -> (w521:string[][])
              n215 = for {
                tunnel: w521 -> [w551] mode=indexing
                tunnel: w525 -> [w556]
                tunnel: w524 -> [w559]
                shift-right: [w558] -> w522
                shift-left: string[][] [] -> [w552]
                stop <- TRUE continue-if-true
                n216 = Index Array(array=w551, index=2) -> (element=w560:string)
                n217 = Empty String/Path?(string/path=w556) -> (empty?=w554:bool)
                n218 = Equal?(x=w556, y=w560) -> (x = y?=w555:bool)
                n219 = Or(x=w554, y=w555) -> (x .or. y?=w553:bool)
                n220 = case shown="True" w553 {
                  tunnel: w551 -> [_ w572]
                  tunnel: w559 -> [_ w567]
                  tunnel: [FALSE w570] -> w550
                  frame False {
                  }
                  frame True {
                    n221 = Index Array(array=w572, index=5) -> (element=w571:string)
                    n222 = Empty String/Path?(string/path=w567) -> (empty?=w568:bool)
                    n223 = Equal?(x=w567, y=w571) -> (x = y?=w569:bool)
                    n224 = Or(x=w568, y=w569) -> (x .or. y?=w570:bool)
                  }
                }
                n225 = case shown="True" w550 {
                  tunnel: w552 -> [w562 w565]
                  tunnel: w551 -> [_ w564]
                  tunnel: [w562 w563] -> w558
                  frame False {
                  }
                  frame True {
                    n226 = Build Array (concatenate)(w565, w564) -> (w563:string[][])
                  }
                }
              }
              n227 = flat-sequence {
                tunnel: w522 -> [w528]
                tunnel: w518 -> [w527]
                tunnel: [w526] -> w519
                tunnel: [w542] -> w520
                tunnel: w519 -> [w541]
                tunnel: w518 -> [w540]
                frame #0 {
                  # "send each element of the array through the TCP connection"
                  n228 = for {
                    tunnel: w528 -> [w531] mode=indexing
                    tunnel: w527 -> [w530]
                    tunnel: [w529] -> w526
                    n229 = for {
                      tunnel: w531 -> [w534] mode=indexing
                      tunnel: w530 -> [w533]
                      tunnel: [w532] -> w529
                      n230 = String Length(string=w534) -> (length=w538:i32)
                      n231 = Number To Decimal String(number=w538, width (-)=i16 10) -> (decimal integer string=w537:string)
                      n232 = TCP Write(connection ID=w533, data in=w537) -> (connection ID out=w535:refnum<k5>, error out=w536:errorcluster)  [unwired: 2 in, 1 out]
                      n233 = TCP Write(connection ID=w535, data in=w534, error in (no error)=w536) -> (error out=w532:errorcluster)  [unwired: 1 in, 2 out]
                    }
                  }
                }
                frame #1 {
                  w544 = "EndOfTx" ("data in")
                  n234 = String Length(string=w544) -> (length=w547:i32)
                  n235 = Number To Decimal String(number=w547, width (-)=i16 10) -> (decimal integer string=w548:string)
                  n236 = TCP Write(connection ID=w540, data in=w548) -> (connection ID out=w545:refnum<k5>, error out=w549:errorcluster)  [unwired: 2 in, 1 out]
                  n237 = TCP Write(connection ID=w545, data in=w544, error in (no error)=w549) -> (error out=w543:errorcluster)  [unwired: 1 in, 2 out]
                  n238 = Merge Errors(w543, w541) -> (w542:errorcluster)
                }
              }
            }
          }
          n239 = case shown="True" w292 {
            tunnel: w283 -> [_ w582]
            tunnel: w282 -> [_ w581]
            tunnel: w281 -> [_ w580]
            tunnel: w247 -> [_ w576]
            tunnel: [errorcluster {"status"=FALSE, "code"=0, "source"=""} ("error IO") w577] -> w280
            frame False {
            }
            frame True {
              # "check each row of the array to see if it matches. If yes, append that row to the result array"
              n240 = local read "Real-time Data from Motes"() -> (w583:string[][])
              n241 = for {
                tunnel: w583 -> [w608] mode=indexing
                tunnel: w582 -> [w614]
                tunnel: w581 -> [w619]
                tunnel: w580 -> [w618]
                shift-right: [w616] -> w578
                shift-left: string[][] [] -> [w609]
                stop <- TRUE continue-if-true
                n242 = Index Array(array=w608, index=2) -> (element=w620:string)
                n243 = Empty String/Path?(string/path=w614) -> (empty?=w612:bool)
                n244 = Equal?(x=w614, y=w620) -> (x = y?=w613:bool)
                n245 = Or(x=w612, y=w613) -> (x .or. y?=w611:bool)
                n246 = case shown="True" w611 {
                  tunnel: w608 -> [_ w640]
                  tunnel: w619 -> [_ w635]
                  tunnel: [FALSE w638] -> w610
                  frame False {
                  }
                  frame True {
                    n247 = Index Array(array=w640, index=1) -> (element=w639:string)
                    n248 = Empty String/Path?(string/path=w635) -> (empty?=w636:bool)
                    n249 = Equal?(x=w635, y=w639) -> (x = y?=w637:bool)
                    n250 = Or(x=w636, y=w637) -> (x .or. y?=w638:bool)
                  }
                }
                n251 = case shown="True" w610 {
                  tunnel: w608 -> [_ w632]
                  tunnel: w618 -> [_ w628]
                  tunnel: [FALSE w627] -> w617
                  frame False {
                  }
                  frame True {
                    n252 = Index Array(array=w632, index=5) -> (element=w631:string)
                    n253 = Equal?(x=w628, y=w631) -> (x = y?=w630:bool)
                    n254 = Empty String/Path?(string/path=w628) -> (empty?=w629:bool)
                    n255 = Or(x=w629, y=w630) -> (x .or. y?=w627:bool)
                  }
                }
                n256 = case shown="True" w617 {
                  tunnel: w609 -> [w622 w625]
                  tunnel: w608 -> [_ w624]
                  tunnel: [w622 w623] -> w616
                  frame False {
                  }
                  frame True {
                    n257 = Build Array (concatenate)(w625, w624) -> (w623:string[][])
                  }
                }
              }
              n258 = flat-sequence {
                tunnel: w578 -> [w586]
                tunnel: w576 -> [w585]
                tunnel: [w584] -> w575
                tunnel: [w598] -> w577
                tunnel: w576 -> [w600]
                tunnel: w575 -> [w599]
                frame #0 {
                  # "send each element of the array through the TCP connection"
                  n259 = for {
                    tunnel: w586 -> [w589] mode=indexing
                    tunnel: w585 -> [w588]
                    tunnel: [w587] -> w584
                    n260 = for {
                      tunnel: w589 -> [w592] mode=indexing
                      tunnel: w588 -> [w591]
                      tunnel: [w590] -> w587
                      n261 = String Length(string=w592) -> (length=w596:i32)
                      n262 = Number To Decimal String(number=w596, width (-)=i16 10) -> (decimal integer string=w595:string)
                      n263 = TCP Write(connection ID=w591, data in=w595) -> (connection ID out=w593:refnum<k5>, error out=w594:errorcluster)  [unwired: 2 in, 1 out]
                      n264 = TCP Write(connection ID=w593, data in=w592, error in (no error)=w594) -> (error out=w590:errorcluster)  [unwired: 1 in, 2 out]
                    }
                  }
                }
                frame #1 {
                  w602 = "EndOfTx" ("data in")
                  n265 = String Length(string=w602) -> (length=w605:i32)
                  n266 = Number To Decimal String(number=w605, width (-)=i16 10) -> (decimal integer string=w606:string)
                  n267 = TCP Write(connection ID=w600, data in=w606) -> (connection ID out=w603:refnum<k5>, error out=w607:errorcluster)  [unwired: 2 in, 1 out]
                  n268 = TCP Write(connection ID=w603, data in=w602, error in (no error)=w607) -> (error out=w601:errorcluster)  [unwired: 1 in, 2 out]
                  n269 = Merge Errors(w601, w599) -> (w598:errorcluster)
                }
              }
            }
          }
          n270 = Merge Errors(w280, w279, w270, w259, w246) -> (w286:errorcluster)
          "error out" <- w286
          n271 = Unbundle By Name(w286) -> ("status"=w285:bool)
        }
      }
      frame Error {
      }
    }
  }
